vi "set_dipole_voltage.vi"(0 "Dipole average settings":T1, 1 "iteration number":i32, 2 "Num files":i32=1) -> ()   [LabVIEW 2018]
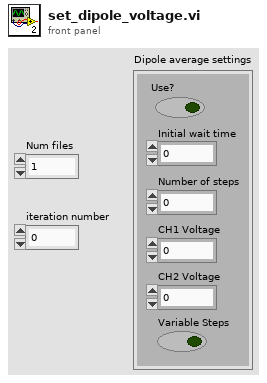
[diagram p1: front panel]
types:
  T1 = cluster{"Initial wait time":dbl, "Number of steps":i32, "CH1 Voltage":dbl, "Use?":bool, "CH2 Voltage":dbl, "Variable Steps":bool}
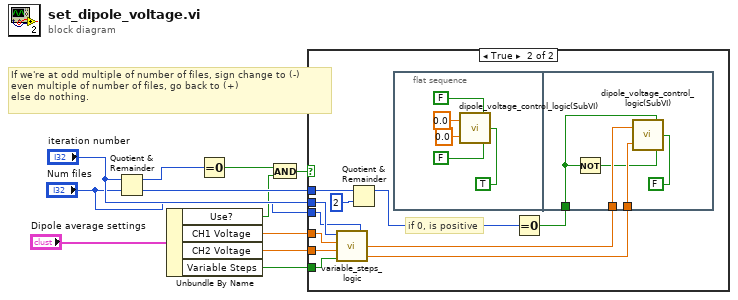
[diagram p0: block diagram]
diagram:
  # "If we're at odd multiple of number of files, sign change to (-)\neven multiple of number of files, go back to (+)\nelse do nothing."
  n1 = Quotient & Remainder(x="iteration number", y="Num files") -> (x-y*floor(x/y)=w9:i32, floor(x/y)=w10:i32)
  n2 = Unbundle By Name("Dipole average settings") -> ("Use?"=w3:bool, "CH1 Voltage"=w7:dbl, "CH2 Voltage"=w6:dbl, "Variable Steps"=w5:bool)
  n3 = Equal To 0?(x=w9) -> (x = 0?=w2:bool)
  n4 = And(x=w2, y=w3) -> (x .and. y?=w4:bool)
  n5 = case shown="True" w4 {
    tunnel: w10 -> [_ w22]
    tunnel: "iteration number" -> [_ w17]
    tunnel: w7 -> [_ w16]
    tunnel: w6 -> [_ w15]
    tunnel: w5 -> [_ w14]
    tunnel: "Num files" -> [_ w12]
    frame False {
    }
    frame True {
      # "if 0, is positive"
      n6 = call "variable_steps_logic.vi"("Num files"=w12, "Variable Steps"=w14, "Voltage 2"=w15, "Voltage 1"=w16, "iteration number"=w17) -> ("Returned Voltage 2"=w18:dbl, "Returned Voltage 1"=w19:dbl)
      n7 = Quotient & Remainder(x=w22, y=2) -> (x-y*floor(x/y)=w21:i32)  [unwired: 1 out]
      n8 = flat-sequence {
        tunnel: w18 -> [w31]
        tunnel: w19 -> [w30]
        tunnel: w20 -> [w28]
        frame #0 {
          n9 = call "dipole_voltage_control_logic(SubVI).vi"("CH1 Voltage"=0.0, "CH2 Voltage"=0.0, "positive"=FALSE, "off"=TRUE, "negative"=FALSE) -> ()
        }
        frame #1 {
          n10 = Not(x=w28) -> (.not. x?=w29:bool)
          n11 = call "dipole_voltage_control_logic(SubVI).vi"("CH1 Voltage"=w30, "CH2 Voltage"=w31, "positive"=w28, "off"=FALSE, "negative"=w29) -> ()
        }
      }
      n12 = Equal To 0?(x=w21) -> (x = 0?=w20:bool)
    }
  }
